vi "FTW-Test-Expressions-Booleanish.vi"() -> (0 "error out":errorcluster)   [LabVIEW 2014]
uses:
  src/core/error/FTW-ERR-ExceptionType.ctl
  src/core/expression/FTW-Expr-BooleanExpressionResult.ctl
  src/core/error/FTW-ERR-ThrowError.vi
  src/core/error/FTW-ERR-NoErrorConstant.vi
  src/core/error/FTW-ERR-CallChain.vi
  src/core/string/FTW-STR-ReplaceWhitespace.vi
  src/core/regex/FTW-Regex.lvclass
panel:
  out "String":string
  out "Array":string[](array[string])
  out "Results":T3(array[cluster])
  out "Lexicon":string="$test == true || $b == false && $c == false"
  out "Capture Groups":string[](array[string])
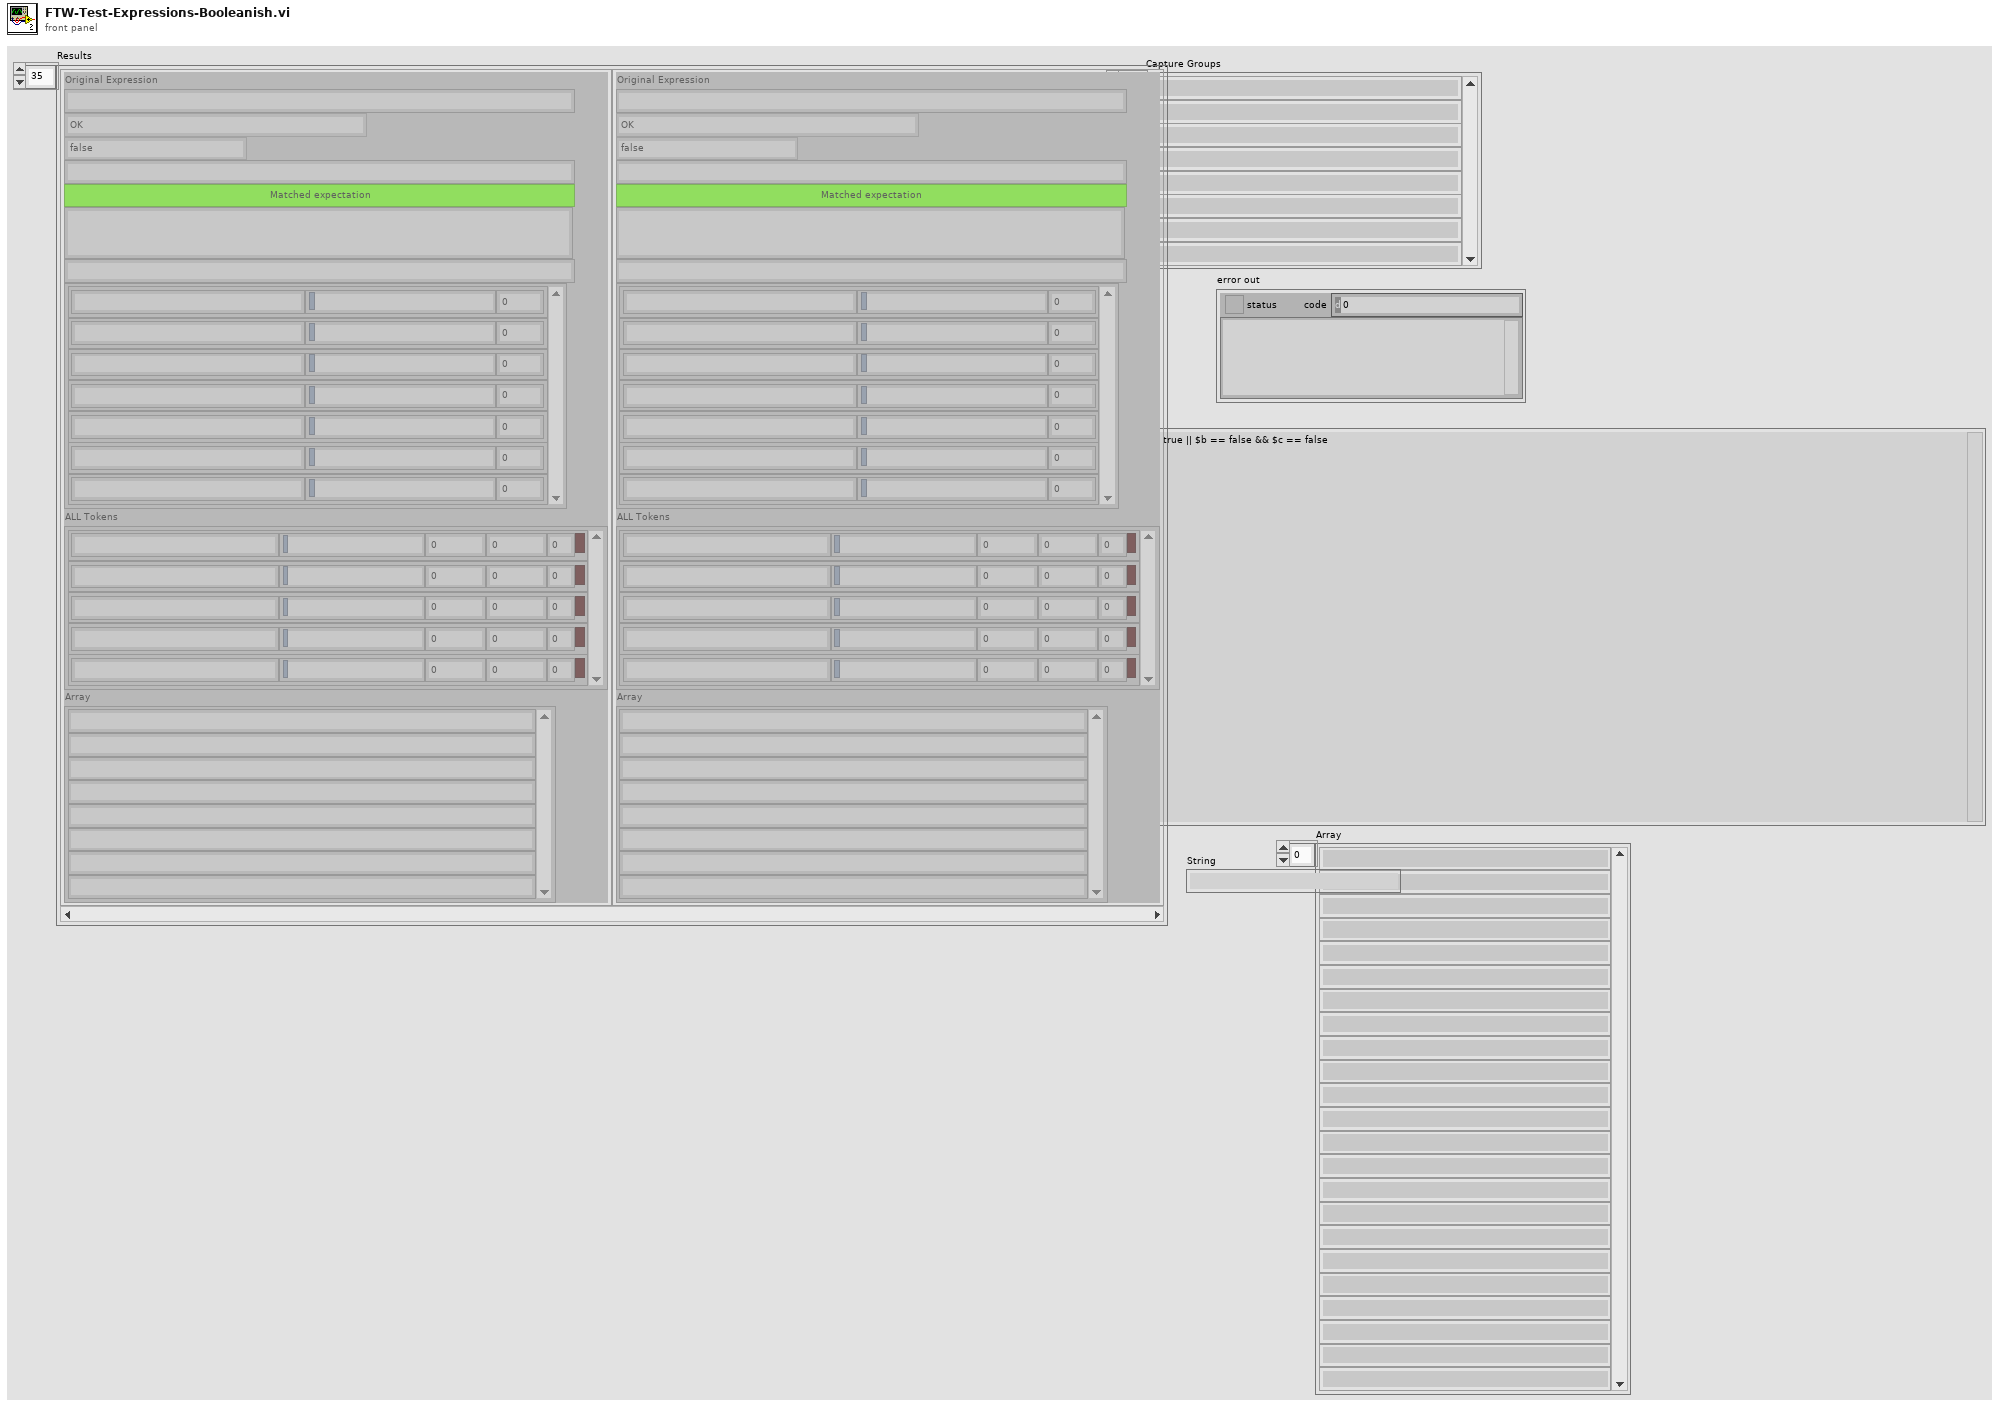
[diagram p1: front panel]
types:
  T1 = typedef "FTW-ERR-ExceptionType.ctl" = enum16{"OK", "Info", "Warning", "Error"}
  T2 = typedef "FTW-Expr-BooleanExpressionResult.ctl" = enum16{"false", "true", "inconclusive"}
  T3 = cluster{"Original Expression":string, "Expression Validity Expectation":T1, "Result":T2, "Expectation":string, "Expectation satisfied?":bool, "Error":string, "Final JSON":string, "Parsed Expression":cluster{string, string, "start_pos":i32}[], "ALL Tokens":cluster{string, string, "prev_pos":i32, "curr_pos":i32, "scope_level":i32, "trimmed?":bool}[], "Array":string[]}[]
  T4 = cluster{"Expression":string, "Expectation":string, "Expression Check":T1, "Value Expectation":T2}[]
  T5 = cluster{"op":cluster{"token":string, "value":string, "subj_start":i32}, "Precedence":i32, "Scope Depth":i32}[]
  T6 = cluster{"token":string, "value":string, "subj_start":i32}[]
  T7 = cluster{"callout_id":i32, "subject_current_pos":i32, "subject_start_match_pos":i32, "cap_top":i32, "cap_last":i32, "patt_pos":i32, "callout_name_index":i32, "callout_name_length":i32}[]
  T8 = cluster{"Text":string, "Expression":string, "Previous Subject Position":i32}
  T9 = cluster{"Text":string, "Expression":string, "Previous Subject Position":i32}[]
  T10 = cluster{cluster{"Text":string, "Expression":string, "Previous Subject Position":i32}, "Precedence":i32, i32}
  T11 = cluster{"op":cluster{"token":string, "value":string, "subj_start":i32}, "Precedence":i32, "Scope Depth":i32}
  T12 = cluster{"token":string, "value":string, "subj_start":i32}
  T13 = cluster{cluster{"Text":string, "Expression":string, "Previous Subject Position":i32}, "default value 1":i32, "Current Scope Depth":i32}
  T14 = cluster{"Text":string, "Expression":string, "subject_current_pos":i32, "Previous Subject Position":i32, "Current Scope Depth":i32, bool}
  T15 = typedef "FTW-JSON-Type.ctl" = enum8{"Not Found", "Object", "Array", "String", "Number", "Boolean", "null"}
  T16 = cluster{"Expression":string, "Expression Check":T1, "Result":T2, "Expectation":string, bool, "source":string, "JSON String (UTF-8)":string, "Reverse Polish Notation Token Stack":cluster{"token":string, "value":string, "subj_start":i32}[], cluster{"Text":string, "Expression":string, "subject_current_pos":i32, "Previous Subject Position":i32, "Current Scope Depth":i32, bool}[], "Try Paths":string[]}
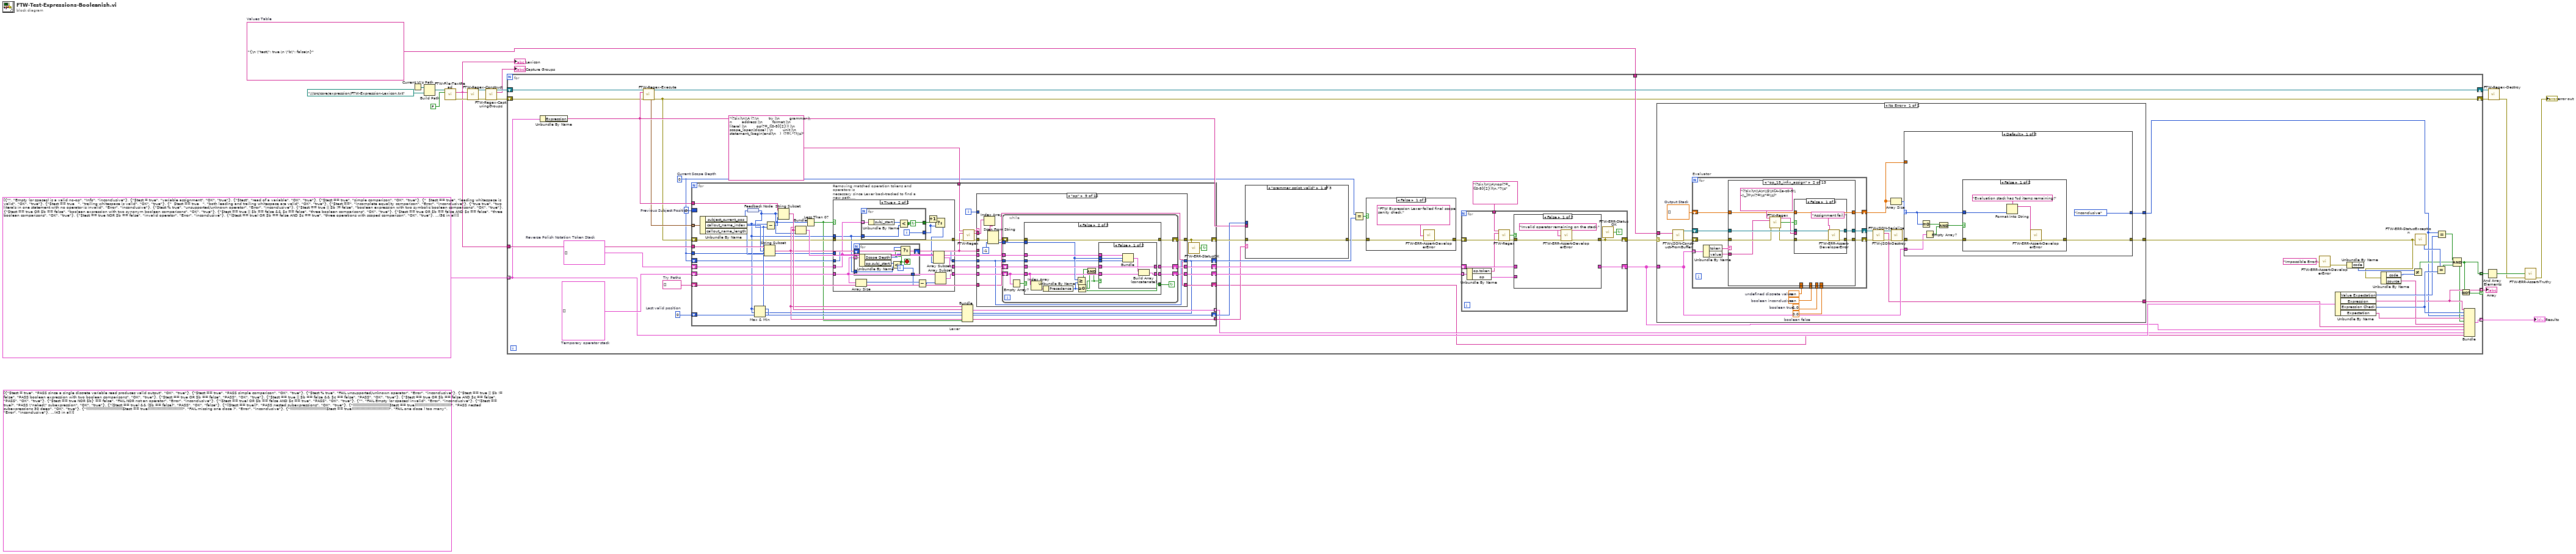
[diagram p0: block diagram]
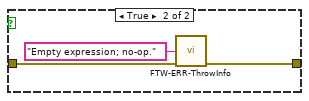
[diagram p2: hidden frame]
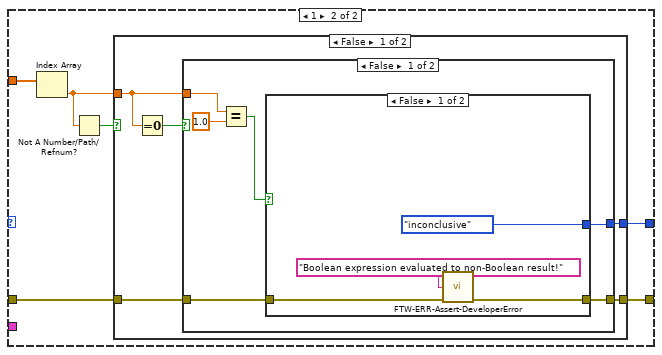
[diagram p3: hidden frame]
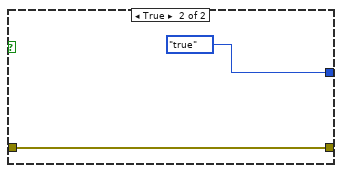
[diagram p4: hidden frame]
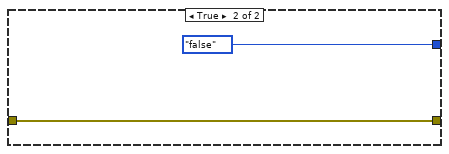
[diagram p5: hidden frame]
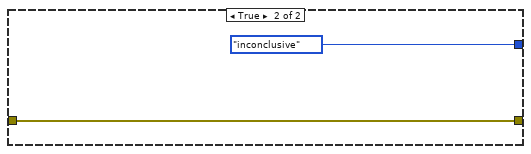
[diagram p6: hidden frame]
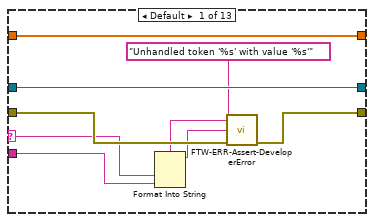
[diagram p7: hidden frame]
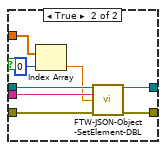
[diagram p8: hidden frame]
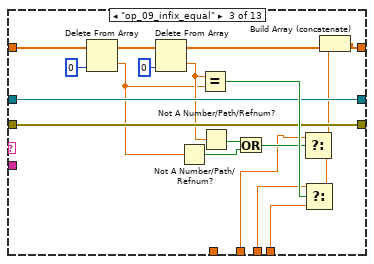
[diagram p9: hidden frame]
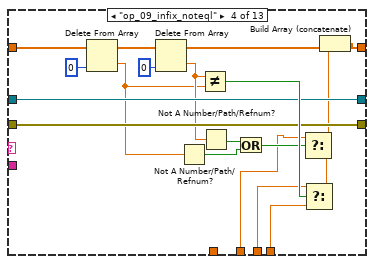
[diagram p10: hidden frame]
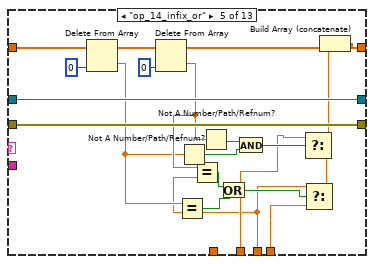
[diagram p11: hidden frame]
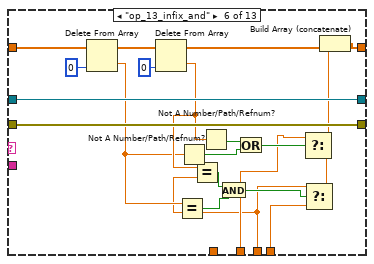
[diagram p12: hidden frame]
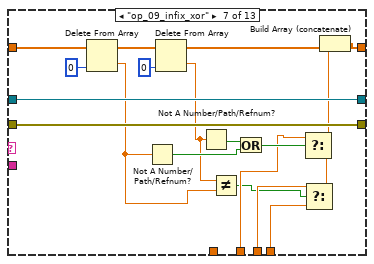
[diagram p13: hidden frame]
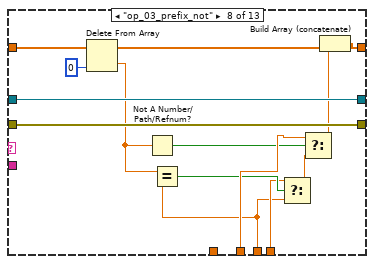
[diagram p14: hidden frame]
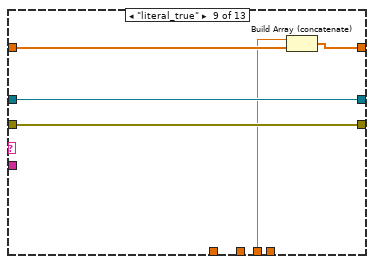
[diagram p15: hidden frame]
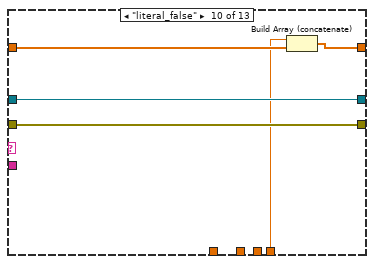
[diagram p16: hidden frame]
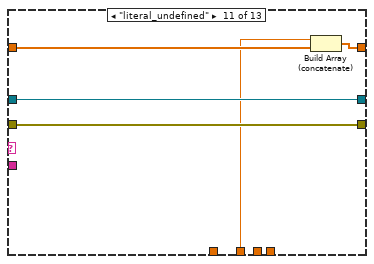
[diagram p17: hidden frame]
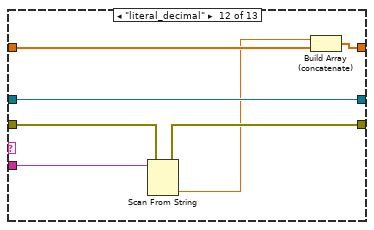
[diagram p18: hidden frame]
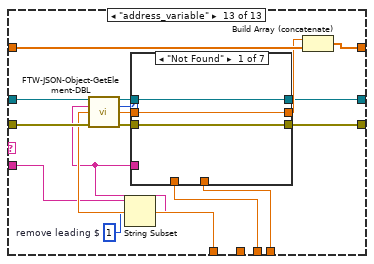
[diagram p19: hidden frame]
diagram:
  (unwired) T4 [{"Expression"="$test = true", "Expectation"="PASS since a single discrete variable read produces valid output", "Expression Check"=enum."OK", "Value Expectation"=enum."true"}, {"Expression"="$test == true", "Expectation"="PASS simple comparison", "Expression Check"=enum."OK", "Value Expectation"=enum."true"}, {"Expression"="$test % true", "Expectation"="FAIL unsupported/unknown operator", "Expression Check"=enum."Error", "Value Expectation"=enum."inconclusive"}, {"Expression"="$test == true || $b != false", "Expectation"="PASS boolean expression with two boolean comparisons", "Expression Check"=enum."OK", "Value Expectation"=enum."true"}, {"Expression"="$test == true OR $b == false", "Expectation"="PASS", "Expression Check"=enum."OK", "Value Expectation"=enum."true"}, {"Expression"="$test == true || $b == false && $c == false", "Expectation"="PASS", "Expression Check"=enum."OK", "Value Expectation"=enum."true"}, {"Expression"="$test == true OR $b == false AND $c == false", "Expectation"="PASS", "Expression Check"=enum."OK", "Value Expectation"=enum."true"}, {"Expression"="$test == true NOR $b} == false", "Expectation"="FAIL NOR not an operator", "Expression Check"=enum."Error", "Value Expectation"=enum."inconclusive"}, {"Expression"="($test == true) OR $b == false AND $c == true", "Expectation"="PASS", "Expression Check"=enum."OK", "Value Expectation"=enum."true"}, {"Expression"="", "Expectation"="FAIL Empty (or spaces) invalid", "Expression Check"=enum."Error", "Value Expectation"=enum."inconclusive"}, {"Expression"="($test == true)", "Expectation"="PASS \"naked\" subexpression", "Expression Check"=enum."OK", "Value Expectation"=enum."true"}, {"Expression"="($test == true) && ($b == false)", "Expectation"="PASS", "Expression Check"=enum."OK", "Value Expectation"=enum."false"}, {"Expression"="(($test == true))", "Expectation"="PASS nested subexpressions", "Expression Check"=enum."OK", "Value Expectation"=enum."true"}, {"Expression"="(((((((((((((((((((((((((((((($test == true))))))))))))))))))))))))))))))", "Expectation"="PASS nested subexpressions 30 deep", "Expression Check"=enum."OK", "Value Expectation"=enum."true"}, {"Expression"="(((((((((((((((((((((((((((((($test == true)))))))))))))))))))))))))))))", "Expectation"="FAIL missing one close )", "Expression Check"=enum."Error", "Value Expectation"=enum."inconclusive"}, {"Expression"="(((((((((((((((((((((((((((((($test == true)))))))))))))))))))))))))))))))", "Expectation"="FAIL one close ) too many", "Expression Check"=enum."Error", "Value Expectation"=enum."inconclusive"}, {"Expression"="true", "Expectation"="PASS plain constant", "Expression Check"=enum."OK", "Value Expectation"=enum."true"}, {"Expression"="False", "Expectation"="PASS plain constant", "Expression Check"=enum."OK", "Value Expectation"=enum."false"}, {"Expression"="ALWAYS AND NEVER", "Expectation"="PASS expression of two boolexpr constants", "Expression Check"=enum."OK", "Value Expectation"=enum."inconclusive"}, {"Expression"="ALWAYS XOR NEVER", "Expectation"="PASS expression of two boolexpr constants", "Expression Check"=enum."OK", "Value Expectation"=enum."inconclusive"}, {"Expression"="(true == true) AND (true EQUALS true) AND (true IS true)", "Expectation"="PASS testing equality operators", "Expression Check"=enum."OK", "Value Expectation"=enum."true"}, {"Expression"="(true != false) AND (true IS NOT false) AND (true <> false)", "Expectation"="PASS testing inequality operators", "Expression Check"=enum."OK", "Value Expectation"=enum."true"}, {"Expression"="(always AND never) XOR (never AND always)", "Expectation"="PASS compound expression of boolexpr constants", "Expression Check"=enum."OK", "Value Expectation"=enum."false"}, {"Expression"="$A==$B", "Expectation"="PASS compare two variables to each other", "Expression Check"=enum."OK", "Value Expectation"=enum."inconclusive"}, {"Expression"="$a!=$b", "Expectation"="PASS since this is a synonym for XOR", "Expression Check"=enum."OK", "Value Expectation"=enum."inconclusive"}, {"Expression"="$A AND $B", "Expectation"="PASS assuming, variables are boolexpr states", "Expression Check"=enum."OK", "Value Expectation"=enum."inconclusive"}, {"Expression"="$a IS true for 3 sec", "Expectation"="SKIP PASS simple timer test", "Expression Check"=enum."OK", "Value Expectation"=enum."inconclusive"}, {"Expression"="$a IS true for 3min", "Expectation"="SKIP PASS no space between timer value and unit", "Expression Check"=enum."OK", "Value Expectation"=enum."inconclusive"}, {"Expression"="$a IS true for 3", "Expectation"="SKIP FAIL no timer units", "Expression Check"=enum."OK", "Value Expectation"=enum."inconclusive"}, {"Expression"="$a IS true   for minute", "Expectation"="SKIP FAIL no timer value", "Expression Check"=enum."OK", "Value Expectation"=enum."inconclusive"}, {"Expression"="$a == true || $b AND $c", "Expectation"="PASS", "Expression Check"=enum."OK", "Value Expectation"=enum."inconclusive"}, {"Expression"="alwaysornever", "Expectation"="FAIL no word boundary on neither operator nor constants", "Expression Check"=enum."OK", "Value Expectation"=enum."inconclusive"}, {"Expression"="always||never", "Expectation"="PASS even though no spaces, the symbolic operator makes a word boundary", "Expression Check"=enum."OK", "Value Expectation"=enum."inconclusive"}, {"Expression"="(($a&&$b) OR ($c&&$d)) AND (($e&&$f) OR ($g&&$h))", "Expectation"="PASS compound expression", "Expression Check"=enum."OK", "Value Expectation"=enum."inconclusive"}, {"Expression"="$a (AND $b)", "Expectation"="FAIL improper placement of parentheses", "Expression Check"=enum."OK", "Value Expectation"=enum."inconclusive"}, {"Expression"="($a)($b)", "Expectation"="FAIL no operator between scopes", "Expression Check"=enum."OK", "Value Expectation"=enum."inconclusive"}, {"Expression"="($a)                   or                 ($b)", "Expectation"="PASS goofy amount of space", "Expression Check"=enum."OK", "Value Expectation"=enum."inconclusive"}, {"Expression"="NOT ALWAYS", "Expectation"="PASS the inversion of a boolexpr constant", "Expression Check"=enum."OK", "Value Expectation"=enum."inconclusive"}, {"Expression"="NOT $a || $b", "Expectation"="PASS even though it could use some parentheses for clarity, this is valid", "Expression Check"=enum."OK", "Value Expectation"=enum."inconclusive"}, {"Expression"="NOT ($a || $b)", "Expectation"="PASS", "Expression Check"=enum."OK", "Value Expectation"=enum."inconclusive"}, {"Expression"="(NOT $a) || $b", "Expectation"="PASS", "Expression Check"=enum."OK", "Value Expectation"=enum."inconclusive"}, {"Expression"="$a && !$b", "Expectation"="PASS", "Expression Check"=enum."OK", "Value Expectation"=enum."inconclusive"}, {"Expression"="IMMEDIATELY", "Expectation"="PASS this is a synonym for ALWAYS", "Expression Check"=enum."OK", "Value Expectation"=enum."inconclusive"}]
  w6 = "{\n \"test\": true,\n \"b\": false\n}"  # Values Table
  n1 = Current VI's Path() -> (path=w17:path)
  n2 = Build Path(base path=w17, name or relative path=path "../../../src/core/expression/FTW-Expression-Lexicon.txt" ("path")) -> (appended path=w15:path)
  n3 = call "FTW-File-TextRead.vi"("Filepath"=w15, "Create if doesn't exist?"=FALSE) -> ("Text"=w18:string, "error out"=w19:errorcluster)  [unwired: 11 in, 1 out]
  "Lexicon" <- w18
  n4 = call "FTW-Regex-Construct.vi"("Regular Expression"=w18, "error in"=w19) -> ("Regex"=w13:refnum<class "FTW-Regex.lvclass">, "error out"=w14:errorcluster)  [unwired: 12 in]
  n5 = call "FTW-Regex-CapturingGroups.vi"("Regex"=w13, "error in"=w14) -> ("Regex out"=w21:refnum<class "FTW-Regex.lvclass">, "Capture Groups"=→"Capture Groups":string[], "error out"=w7:errorcluster)  [unwired: 11 in]
  n6 = for {
    tunnel: w18 -> [w69]
    shift-right: [w54] -> w11
    shift-left: w21 -> [w70]
    tunnel: T4 [{"Expression"="", "Expectation"="Empty (or spaces) is a valid no-op", "Expression Check"=enum."Info", "Value Expectation"=enum."inconclusive"}, {"Expression"="$test = true", "Expectation"="variable assignment", "Expression Check"=enum."OK", "Value Expectation"=enum."true"}, {"Expression"="$test", "Expectation"="read of a variable", "Expression Check"=enum."OK", "Value Expectation"=enum."true"}, {"Expression"="$test == true", "Expectation"="simple comparison", "Expression Check"=enum."OK", "Value Expectation"=enum."true"}, {"Expression"="  $test == true", "Expectation"="leading whitespace is valid", "Expression Check"=enum."OK", "Value Expectation"=enum."true"}, {"Expression"="$test == true   ", "Expectation"="trailing whitespace is valid", "Expression Check"=enum."OK", "Value Expectation"=enum."true"}, {"Expression"="  $test == true   ", "Expectation"="both leading and trailing whitespace are valid", "Expression Check"=enum."OK", "Value Expectation"=enum."true"}, {"Expression"="$test ==", "Expectation"="incomplete equality comparison", "Expression Check"=enum."Error", "Value Expectation"=enum."inconclusive"}, {"Expression"="true true", "Expectation"="two literals in one statement with no operator is invalid", "Expression Check"=enum."Error", "Value Expectation"=enum."inconclusive"}, {"Expression"="$test % true", "Expectation"="unsupported/unknown operator", "Expression Check"=enum."Error", "Value Expectation"=enum."inconclusive"}, {"Expression"="$test == true || $b != false", "Expectation"="boolean expression with two symbolic boolean comparisons", "Expression Check"=enum."OK", "Value Expectation"=enum."true"}, {"Expression"="$test == true OR $b == false", "Expectation"="boolean expression with two synonym boolean comparisons", "Expression Check"=enum."OK", "Value Expectation"=enum."true"}, {"Expression"="$test == true || $b == false && $c == false", "Expectation"="three boolean comparisons", "Expression Check"=enum."OK", "Value Expectation"=enum."true"}, {"Expression"="$test == true OR $b == false AND $c == false", "Expectation"="three boolean comparisons", "Expression Check"=enum."OK", "Value Expectation"=enum."true"}, {"Expression"="$test == true NOR $b == false", "Expectation"="invalid operator", "Expression Check"=enum."Error", "Value Expectation"=enum."inconclusive"}, {"Expression"="($test == true) OR $b == false AND $c == true", "Expectation"="three operations with scoped comparison", "Expression Check"=enum."OK", "Value Expectation"=enum."true"}, {"Expression"="$test OR ($test == false)", "Expectation"="variable comparison with subexpression", "Expression Check"=enum."OK", "Value Expectation"=enum."true"}, {"Expression"="($test == true)", "Expectation"="superfluous subexpression", "Expression Check"=enum."OK", "Value Expectation"=enum."true"}, {"Expression"="($test == true) && ($b == false)", "Expectation"="operation on two subexpressions", "Expression Check"=enum."OK", "Value Expectation"=enum."true"}, {"Expression"="(($test == true))", "Expectation"="nested subexpressions", "Expression Check"=enum."OK", "Value Expectation"=enum."true"}, {"Expression"="(((((((((((((((((((((((((((((($test == true))))))))))))))))))))))))))))))", "Expectation"="PASS nested subexpressions 30 deep", "Expression Check"=enum."OK", "Value Expectation"=enum."true"}, {"Expression"="(((((((((((((((((((((((((((((($test == true)))))))))))))))))))))))))))))", "Expectation"="missing one close )", "Expression Check"=enum."Error", "Value Expectation"=enum."inconclusive"}, {"Expression"="(((((((((((((((((((((((((((((($test == true)))))))))))))))))))))))))))))))", "Expectation"="one close ) too many", "Expression Check"=enum."Error", "Value Expectation"=enum."inconclusive"}, {"Expression"="true", "Expectation"="plain constant", "Expression Check"=enum."OK", "Value Expectation"=enum."true"}, {"Expression"="False", "Expectation"="plain constant", "Expression Check"=enum."OK", "Value Expectation"=enum."false"}, {"Expression"="true XOR false", "Expectation"="expression of two boolexpr constants", "Expression Check"=enum."OK", "Value Expectation"=enum."true"}, {"Expression"="(true == true) AND (true EQUALS true) AND (true IS true)", "Expectation"="testing equality operators", "Expression Check"=enum."OK", "Value Expectation"=enum."true"}, {"Expression"="(true != false) AND (true IS NOT false) AND (true <> false)", "Expectation"="testing inequality operators", "Expression Check"=enum."OK", "Value Expectation"=enum."true"}, {"Expression"="(true AND false) XOR (false AND true)", "Expectation"="compound expression of boolexpr constants", "Expression Check"=enum."OK", "Value Expectation"=enum."false"}, {"Expression"="$A==$B", "Expectation"="compare two variables to each other", "Expression Check"=enum."OK", "Value Expectation"=enum."inconclusive"}, {"Expression"="$a!=$b", "Expectation"="synonym for XOR", "Expression Check"=enum."OK", "Value Expectation"=enum."inconclusive"}, {"Expression"="$A AND $B", "Expectation"="AND two variables", "Expression Check"=enum."OK", "Value Expectation"=enum."inconclusive"}, {"Expression"="$test == ture", "Expectation"="common misspelling of \"true\" is invalid", "Expression Check"=enum."Error", "Value Expectation"=enum."inconclusive"}, {"Expression"="%test == flase", "Expectation"="common misspelling of \"false\" is invalid", "Expression Check"=enum."Error", "Value Expectation"=enum."inconclusive"}, {"Expression"="$test == tru", "Expectation"="incomplete literal \"true\"", "Expression Check"=enum."Error", "Value Expectation"=enum."inconclusive"}, {"Expression"="$test == truee", "Expectation"="extra 'e' in literal \"true\"", "Expression Check"=enum."Error", "Value Expectation"=enum."inconclusive"}, {"Expression"="$test == true!", "Expectation"="unary operator in wrong location", "Expression Check"=enum."Error", "Value Expectation"=enum."inconclusive"}, {"Expression"="$a == true || $b AND $c", "Expectation"="mix of symbolic and synonym operators", "Expression Check"=enum."OK", "Value Expectation"=enum."inconclusive"}, {"Expression"="falseortrue", "Expectation"="invalid without word boundary between operator and literals", "Expression Check"=enum."Error", "Value Expectation"=enum."inconclusive"}, {"Expression"="false||true", "Expectation"="even though no spaces, the symbolic operator makes a word boundary", "Expression Check"=enum."OK", "Value Expectation"=enum."true"}, {"Expression"="(($a&&$b) OR ($c&&$d)) AND (($e&&$f) OR ($g&&$h))", "Expectation"="compound scoped expression", "Expression Check"=enum."OK", "Value Expectation"=enum."inconclusive"}, {"Expression"="$a (AND $b)", "Expectation"="improper placement of parentheses", "Expression Check"=enum."Error", "Value Expectation"=enum."inconclusive"}, {"Expression"="($a)($b)", "Expectation"="no operator between scopes", "Expression Check"=enum."Error", "Value Expectation"=enum."inconclusive"}, {"Expression"="($a)                   or                 ($b)", "Expectation"="goofy but valid amount of space", "Expression Check"=enum."OK", "Value Expectation"=enum."false"}, {"Expression"="NOT $a || $b", "Expectation"="valid, but could use some parentheses for clarity, since precedence applies to first operand and not the result of the operation", "Expression Check"=enum."OK", "Value Expectation"=enum."false"}, {"Expression"="$b || NOT $a", "Expectation"="valid", "Expression Check"=enum."OK", "Value Expectation"=enum."false"}, {"Expression"="$b||!$a", "Expectation"="could use some whitespace, but valid use of symbolic operators", "Expression Check"=enum."OK", "Value Expectation"=enum."false"}, {"Expression"="NOT ($a || $b)", "Expectation"="valid", "Expression Check"=enum."OK", "Value Expectation"=enum."true"}, {"Expression"="(NOT $a) || $b", "Expectation"="valid", "Expression Check"=enum."OK", "Value Expectation"=enum."false"}, {"Expression"="!($a||$b)", "Expectation"="valid", "Expression Check"=enum."OK", "Value Expectation"=enum."true"}, {"Expression"="$a && !$b", "Expectation"="valid", "Expression Check"=enum."OK", "Value Expectation"=enum."inconclusive"}, {"Expression"="! ($test = false)", "Expectation"="assignment in the middle of a statement", "Expression Check"=enum."OK", "Value Expectation"=enum."true"}, {"Expression"="$b | true", "Expectation"="unsupported operator `|`", "Expression Check"=enum."Error", "Value Expectation"=enum."inconclusive"}, {"Expression"="$b & true", "Expectation"="unsupported operator `&`", "Expression Check"=enum."Error", "Value Expectation"=enum."inconclusive"}, {"Expression"="$b IS NOT true", "Expectation"="inequality on boolean", "Expression Check"=enum."OK", "Value Expectation"=enum."true"}, {"Expression"="$b IS NOT NOT false", "Expectation"="inequality on inverted boolean", "Expression Check"=enum."OK", "Value Expectation"=enum."true"}] -> [w52] mode=indexing
    tunnel: [w53] -> w10 mode=indexing
    tunnel: [w31] -> w9 mode=indexing
    tunnel: w6 -> [w41]
    shift-right: [w39] -> w5
    shift-left: w7 -> [w43]
    tunnel: [w32] -> w4 mode=indexing if=w30
    w27 = 0  # Previous Subject Position
    w29 = string[] []  # Try Paths
    w57 = 0  # Last valid position
    w23 = 0  # Current Scope Depth
    w66 = T5 []  # Temporary operator stack
    w67 = T6 []  # Reverse Polish Notation Token Stack
    n7 = Unbundle By Name(w52) -> ("Expression"=w51:string)
    n8 = call "FTW-Regex-Execute.vi"("Regex"=w70, "Subject String"=w51, "error in"=w43) -> ("Regex out"=w54:refnum<class "FTW-Regex.lvclass">, "Callouts"=w40:T7, "error out"=w39:errorcluster)  [unwired: 7 in, 3 out]
    n9 = for "Lexer" {
      tunnel: "(?six)\n\\A (?:\n        try |\n        grammar |\n        address |\n        format |\n        literal |\n        op(?=_([0-9]{2})) |\n        scope_(open|close) | \n        unit |\n        statement_(begin|end)\n   )  (?=(.*?)\\z)" -> [w428]
      shift-right: [w425] -> w58
      shift-left: w67 -> [w403]
      shift-right: [w423] -> w60
      shift-left: w39 -> [w401]
      shift-right: [w421] -> w65
      shift-left: w66 -> [w404]
      shift-right: [w393] -> w63
      shift-left: w23 -> [w397]
      tunnel: w40 -> [w418] mode=indexing
      tunnel: w51 -> [w420]
      tunnel: [w411] -> w42 mode=indexing
      shift-right: [w416] -> w56
      shift-left: w57 -> [w417]
      tunnel: [w409] -> w55
      tunnel: w69 -> [w415]
      shift-right: [w407] -> w28
      shift-left: w29 -> [w408]
      border: w27 -> [_]
      tunnel: w23 -> [w395]
      i -> [w419]
      stop <- w422 continue-if-true
      n10 = Unbundle By Name(w418) -> ("subject_current_pos"=w398:i32, "callout_name_index"=w414:i32, "callout_name_length"=w413:i32)
      n11 = feedback-in #1(w398) -> ()
      n12 = feedback #1() -> (w406:i32)
      n13 = Max & Min(x=w398, y=w417) -> (max(x,y)=w416:i32)  [unwired: 1 out]
      n14 = String Subset(string=w415, offset (0)=w414, length (rest)=w413) -> (substring=w409:string)
      n15 = Subtract(x=w398, y=w406) -> (x-y=w405:i32)
      n16 = String Subset(string=w420, offset (0)=w406, length (rest)=w405) -> (substring=w410:string)
      n17 = Bundle("Text"=w409, "Expression"=w410, "Previous Subject Position"=w406) -> (w412:T8)  [unwired: 1 in]
      n18 = Less Than 0?(x=w405) -> (x < 0?=w394:bool)
      n19 = case "Removing matched operation tokens and operators is \nnecessary since Lexer back-tracked to find a new path,\nnot having found complete grammar of a valid expression" shown="True" w394 {
        tunnel: w404 -> [w431 w436]
        tunnel: w403 -> [w432 w446]
        tunnel: [w430 w447] -> w402
        tunnel: w401 -> [w430 w447]
        tunnel: [w432 w445] -> w400
        tunnel: [w431 w444] -> w399
        tunnel: w398 -> [_ w443]
        tunnel: w397 -> [w429 w437]
        tunnel: [w429 w442] -> w396
        tunnel: w395 -> [_ _]
        frame False {
        }
        frame True {
          n20 = for {
            tunnel: w436 -> [w455] mode=indexing
            tunnel: w443 -> [w453]
            shift-right: [w450] -> w442
            shift-left: w437 -> [w451]
            tunnel: [w448] -> w433
            i -> [w448]
            stop <- w449 stop-if-true
            n21 = Unbundle By Name(w455) -> ("Scope Depth"=w452:i32, "op.subj_start"=w454:i32)
            n22 = Less?(x=w454, y=w453) -> (x < y?=w449:bool)
            n23 = Select(t=w451, s=w449, f=w452) -> (s? t:f=w450:i32)
          }
          n24 = Array Size(array=w436) -> (size(s)=w435:i32)
          n25 = for {
            tunnel: w446 -> [w460] mode=indexing
            tunnel: w443 -> [w458]
            tunnel: [w457] -> w439
            tunnel: [w456] -> w441
            i -> [w457]
            stop <- w456 continue-if-true
            n26 = Unbundle By Name(w460) -> ("subj_start"=w459:i32)
            n27 = Less?(x=w459, y=w458) -> (x < y?=w456:bool)
          }
          n28 = Subtract(x=w435, y=w433) -> (x-y=w434:i32)
          n29 = Increment(x=w439) -> (x+1=w438:i32)
          n30 = Select(t=w438, s=w441, f=w439) -> (s? t:f=w440:i32)
          n31 = Array Subset(array=w446, length=w440) -> (w445:T6)  [unwired: 1 in]
          n32 = Array Subset(array=w436, length=w434) -> (w444:T5)  [unwired: 1 in]
        }
      }
      n33 = call "FTW-Regex.vi"("Regular Expression"=w428, "Input String"=w409, "error in"=w402) -> ("Match"=w427:string, "Submatches"=w426:string[], "error out"=w424:errorcluster)  [unwired: 8 in, 2 out]
      n34 = case shown="\"op\"" w427 {
        tunnel: w426 -> [_ _ _ _ w493 _ _ _ w568 _ _ _]
        tunnel: w412 -> [_ w476 w483 _ _ _ w510 w520 w569 _ _ _]
        tunnel: w400 -> [w467 w475 w482 w488 w497 w504 w513 w524 w573 w629 w634 w639]
        tunnel: [w467 w474 w481 w488 w497 w504 w513 w522 w574 w629 w634 w639] -> w425
        tunnel: [w468 w473 w480 w487 w496 w501 w514 w519 w571 w630 w635 w640] -> w423
        tunnel: w424 -> [w469 w473 w480 w487 w496 w501 w514 w518 w578 w630 w635 w640]
        tunnel: [w466 w472 w479 w486 w495 w503 w511 w521 w570 w628 w633 w638] -> w421
        tunnel: w399 -> [w466 w472 w479 w486 w495 w503 w512 w523 w575 w628 w633 w638]
        tunnel: w409 -> [w463 _ _ _ w489 w498 _ _ _ _ _ _]
        tunnel: w396 -> [w462 w471 w478 w485 w494 w502 w508 w517 w566 w627 w632 w637]
        tunnel: [w462 w471 w478 w485 w494 w502 w507 w516 w566 w627 w632 w637] -> w393
        tunnel: w419 -> [_ _ _ _ _ _ _ _ _ _ _ _]
        tunnel: w408 -> [w461 w470 w477 w484 w491 w500 w505 w515 w565 w626 w631 w636]
        tunnel: [w461 w470 w477 w484 w490 w499 w505 w515 w565 w626 w631 w636] -> w407
        frame Default {
          n35 = Format Into String(format string="Bug in the FTW evaluation compiler! Unknown token: \"%s\"" ("Reason this error should never happen"), w463) -> (resulting string=w464:string)  [unwired: 2 in, 1 out]
          n36 = call "FTW-ERR-Assert-DeveloperError.vi"("Reason this error should never happen"=w464, "error in"=w469) -> ("error out"=w468:errorcluster)  [unwired: 13 in]
        }
        frame "literal" {
          n37 = Build Array (concatenate)(w475, w476) -> (w474:T9)
        }
        frame "address" {
          n38 = Build Array (concatenate)(w482, w483) -> (w481:T9)
        }
        frame "format" {
          # "Format matches are included in the\ncallout array purely to maintain match position\nof tokens."
        }
        frame "try" {
          # "Format matches are included in the\ncallout array purely to maintain match position\nof tokens."
          n39 = Index Array(array=w493) -> (element=→"String":string)  [unwired: 1 in]
          n40 = Build Array (concatenate)(w491, w489) -> (w490:string[])
        }
        frame "grammar" {
          # "Grammar matches are included in the\ncallout array in order to maintain match position\nof tokens and to validate grammar."
          n41 = Build Array (concatenate)(w500, w498) -> (w499:string[])
        }
        frame "scope_open" {
          w506 = -1  # Precedence
          n42 = Increment(x=w508) -> (x+1=w507:i32)
          n43 = Bundle(w510, "Precedence"=w506, w507) -> (w509:T10)  [unwired: 1 in]
          n44 = Build Array (concatenate)(w509, w512) -> (w511:T5)
        }
        frame "scope_close" {
          n45 = while {
            shift-right: [w530] -> w519
            shift-left: w518 -> [w531]
            shift-right: [w539] -> w522
            shift-left: w524 -> [w538]
            shift-right: [w537] -> w521
            shift-left: w523 -> [w536]
            tunnel: w520 -> [_]
            shift-right: [w527] -> w516
            shift-left: w517 -> [w526]
            stop <- w528 continue-if-true
            n46 = Delete From Array(array=w536, index=0) -> (deleted portion=w534:T11, array with subset deleted=w532:T5)  [unwired: 1 in]
            n47 = Unbundle By Name(w534) -> ("Scope Depth"=w525:i32, "op"=w529:T12, "op.token"=w533:string)
            n48 = case shown="Default" w533 {
              tunnel: [w548 w560] -> w539
              tunnel: w538 -> [w547 w560]
              tunnel: [w544 w559] -> w537
              tunnel: w532 -> [w544 w559]
              tunnel: w531 -> [w545 w555]
              tunnel: [w542 w554] -> w530
              tunnel: w529 -> [w546 _]
              tunnel: [w541 _] -> w528
              tunnel: [w540 w558] -> w527
              tunnel: w526 -> [w540 w556]
              tunnel: w525 -> [_ w557]
              frame Default {
                n49 = Empty Array?(array=w544) -> (empty?=w543:bool)
                n50 = case shown="True" w543 {
                  tunnel: w545 -> [w549 w552]
                  tunnel: [w549 w550] -> w542
                  frame False {
                  }
                  frame True {
                    n51 = call "FTW-ERR-Assert-DeveloperError.vi"("Reason this error should never happen"="Mismatched scope", "error in"=w552) -> ("error out"=w550:errorcluster)  [unwired: 13 in]
                  }
                }
                n52 = Build Array (concatenate)(w547, w546) -> (w548:T6)
                n53 = call "FTW-ERR-StatusOK.vi"("error to check"=w542) -> ("Status OK?"=w541:bool)
              }
              frame "scope_open" {
                # "Found it the matching\nscope_open token;\nsilently discard it."
                n54 = Not Equal?(x=w557, y=w556) -> (x != y?=w553:bool)
                n55 = case shown="True" w553 {
                  tunnel: w555 -> [w561 w564]
                  tunnel: [w561 w562] -> w554
                  frame False {
                  }
                  frame True {
                    n56 = call "FTW-ERR-Assert-DeveloperError.vi"("Reason this error should never happen"="Mismatched scope level", "error in"=w564) -> ("error out"=w562:errorcluster)  [unwired: 13 in]
                  }
                }
                n57 = Decrement(x=w556) -> (x-1=w558:i32)
              }
            }
          }
        }
        frame "op" {
          n58 = Index Array(array=w568) -> (element=w567:string)  [unwired: 1 in]
          n59 = Scan From String(input string=w567, error in=w578, default 1=-1 ("default value 1")) -> (error out=w572:errorcluster, output 1=w576:i32)  [unwired: 2 in, 2 out]
          n60 = while {
            tunnel: w576 -> [w584]
            shift-right: [w580] -> w571
            shift-left: w572 -> [w579]
            shift-right: [w589] -> w574
            shift-left: w573 -> [w588]
            shift-right: [w587] -> w570
            shift-left: w575 -> [w586]
            tunnel: w569 -> [w585]
            tunnel: w566 -> [w583]
            stop <- w581 continue-if-true
            n61 = Empty Array?(array=w586) -> (empty?=w582:bool)
            n62 = case shown="False" w582 {
              tunnel: [w598 w611] -> w589
              tunnel: w588 -> [w598 w610]
              tunnel: [w597 w609] -> w587
              tunnel: w586 -> [w596 w605]
              tunnel: w585 -> [w595 w608]
              tunnel: w584 -> [w594 w607]
              tunnel: w583 -> [w593 w606]
              tunnel: [FALSE w599] -> w581
              tunnel: [w590 w603] -> w580
              tunnel: w579 -> [w590 w603]
              frame True {
                n63 = Bundle(w595, "default value 1"=w594, "Current Scope Depth"=w593) -> (w592:T13)  [unwired: 1 in]
                n64 = Build Array (concatenate)(w592, w596) -> (w597:T5)
              }
              frame False {
                n65 = Index Array(array=w605) -> (element=w604:T11)  [unwired: 1 in]
                n66 = Unbundle By Name(w604) -> ("Precedence"=w602:i32)
                n67 = Greater Or Equal?(x=w607, y=w602) -> (x >= y?=w601:bool)
                n68 = Greater Or Equal To 0?(x=w602) -> (x >= 0?=w600:bool)
                n69 = And(x=w601, y=w600) -> (x .and. y?=w599:bool)
                n70 = case shown="False" w599 {
                  tunnel: [w618 w624] -> w611
                  tunnel: w610 -> [w618 w625]
                  tunnel: [w616 w619] -> w609
                  tunnel: w605 -> [w617 w620]
                  tunnel: w608 -> [w615 _]
                  tunnel: w607 -> [w614 _]
                  tunnel: w606 -> [w612 _]
                  frame False {
                    n71 = Bundle(w615, "default value 1"=w614, "Current Scope Depth"=w612) -> (w613:T13)  [unwired: 1 in]
                    n72 = Build Array (concatenate)(w613, w617) -> (w616:T5)
                  }
                  frame True {
                    n73 = Delete From Array(array=w620, index=0) -> (deleted portion=w622:T11, array with subset deleted=w619:T5)  [unwired: 1 in]
                    n74 = Unbundle(w622) -> ("op"=w621:T12)  [unwired: 2 out]
                    n75 = Build Array (concatenate)(w625, w621) -> (w624:T6)
                  }
                }
              }
            }
          }
        }
        frame "unit" {
        }
        frame "statement_begin" {
        }
        frame "statement_end" {
        }
      }
      n76 = Bundle("Text"=w409, "Expression"=w410, "subject_current_pos"=w398, "Previous Subject Position"=w406, "Current Scope Depth"=w393, w394) -> (w411:T14)  [unwired: 1 in]
      n77 = call "FTW-ERR-StatusOK.vi"("error to check"=w423) -> ("Status OK?"=w422:bool)
    }
    n78 = case shown="\"grammar_script_valid\"" w55 {
      tunnel: [w359 w361 w370] -> w59
      tunnel: w60 -> [w359 w362 w369]
      tunnel: w56 -> [_ _ w365]
      tunnel: w51 -> [_ _ w366]
      frame "grammar_script_valid" {
      }
      frame Default {
        n79 = call "FTW-ERR-Assert-DeveloperError.vi"("Reason this error should never happen"="Bogus lexing regex.", "error in"=w362) -> ("error out"=w361:errorcluster)  [unwired: 13 in]
      }
      frame "grammar_script_invalid" {
        n80 = String Subset(string=w366, offset (0)=w365, length (rest)=8 ("length (rest)")) -> (substring=w363:string)
        n81 = Format Into String(format string="Syntax error near character position %d beginning with \"%s\"" ("Error Message"), w365, w363) -> (resulting string=w367:string)  [unwired: 2 in, 1 out]
        n82 = call "FTW-ERR-ThrowGenericError.vi"("Error Message"=w367, "error in"=w369) -> ("error out"=w370:errorcluster)  [unwired: 13 in]
      }
    }
    n83 = Equal?(x=w23, y=w63) -> (x = y?=w62:bool)
    n84 = case shown="False" w62 {
      tunnel: w59 -> [w372 w374]
      tunnel: [w371 w374] -> w61
      frame False {
        n85 = call "FTW-ERR-Assert-DeveloperError.vi"("Reason this error should never happen"="FTW Expression Lexer failed final scope sanity check.", "error in"=w372) -> ("error out"=w371:errorcluster)  [unwired: 13 in]
      }
      frame True {
      }
    }
    n86 = for {
      tunnel: w65 -> [w385] mode=indexing
      shift-right: [w376] -> w33
      shift-left: w61 -> [w384]
      tunnel: "(?six)\n\\A\nop(?=_([0-9]{2}))\n.*?\\z" ("Regular Expression") -> [w383]
      shift-right: [w378] -> w25
      shift-left: w58 -> [w379]
      stop <- w375 continue-if-true
      n87 = Unbundle By Name(w385) -> ("op.token"=w377:string, "op"=w380:T12)
      n88 = call "FTW-Regex.vi"("Regular Expression"=w383, "Input String"=w377, "error in"=w384) -> ("Match Found?"=w382:bool, "error out"=w381:errorcluster)  [unwired: 8 in, 3 out]
      n89 = case shown="False" w382 {
        tunnel: w381 -> [w388 w392]
        tunnel: [w386 w392] -> w376
        tunnel: w380 -> [_ w391]
        tunnel: w379 -> [_ w390]
        tunnel: [_ w389] -> w378
        frame False {
          n90 = call "FTW-ERR-Assert-DeveloperError.vi"("Reason this error should never happen"="Invalid operator remaining on the stack.", "error in"=w388) -> ("error out"=w386:errorcluster)  [unwired: 13 in]
        }
        frame True {
          n91 = Build Array (concatenate)(w390, w391) -> (w389:T6)
        }
      }
      n92 = call "FTW-ERR-StatusOK.vi"("error to check"=w376) -> ("Status OK?"=w375:bool)
    }
    n93 = case shown="No Error" w33 {
      selector: w33 -> [w82 w358]
      tunnel: [w78 w358] -> w24
      tunnel: w25 -> [w76 _]
      tunnel: w41 -> [w83 _]
      tunnel: [w77 FTW-Expr-BooleanExpressionResult."inconclusive" ("Result")] -> w26
      tunnel: [w71 "" ("JSON String (UTF-8)")] -> w22
      frame No Error {
        w84 = nan  # undefined discrete value
        w85 = nan  # boolean inconclusive
        w86 = 1.0  # boolean true
        w87 = 0.0  # boolean false
        w88 = dbl[] []  # Output Stack
        n94 = call "FTW-JSON-Construct-FromBuffer.vi"("JSON String (UTF-8)"=w83, "error in"=w82) -> ("JSON Object"=w89:refnum<data-value>, "error out"=w90:errorcluster)  [unwired: 12 in]
        n95 = for "Evaluator" {
          tunnel: w76 -> [w146] mode=indexing
          shift-right: [w143] -> w80
          shift-left: w88 -> [w144]
          shift-right: [w141] -> w75
          shift-left: w89 -> [w142]
          shift-right: [w139] -> w73
          shift-left: w90 -> [w140]
          tunnel: w87 -> [w138]
          tunnel: w86 -> [w137]
          tunnel: w85 -> [w136]
          tunnel: w84 -> [w135]
          n96 = Unbundle By Name(w146) -> ("token"=w145:string, "value"=w134:string)
          n97 = case shown="\"op_15_infix_assign\"" w145 {
            selector: w145 -> [w148 _ _ _ _ _ _ _ _ _ _ _ _]
            tunnel: w144 -> [w154 w156 w195 w214 w235 w256 w275 w289 w294 w299 w304 w311 w328]
            tunnel: [w154 w156 w189 w208 w230 w251 w270 w287 w293 w298 w303 w310 w327] -> w143
            tunnel: w142 -> [w153 w164 w188 w207 w229 w250 w269 w286 w292 w297 w302 w309 w326]
            tunnel: [w153 w163 w188 w207 w229 w250 w269 w286 w292 w297 w302 w309 w318] -> w141
            tunnel: w140 -> [w152 w161 w187 w206 w228 w249 w268 w285 w291 w296 w301 w307 w325]
            tunnel: [w151 w162 w187 w206 w228 w249 w268 w285 w291 w296 w301 w306 w317] -> w139
            tunnel: w134 -> [w147 w158 _ _ _ _ _ _ _ _ _ w308 w313]
            tunnel: w138 -> [_ _ w179 w198 w222 w243 w262 w278 _ w295 _ _ w315]
            tunnel: w137 -> [_ _ w178 w197 w217 w238 w260 w277 w290 _ _ _ w316]
            tunnel: w136 -> [_ _ w177 w196 w221 w242 w261 w283 _ _ w300 _ _]
            tunnel: w135 -> [_ _ _ _ _ _ _ _ _ _ _ _ w324]
            frame Default {
              n98 = Format Into String(format string="Unhandled token '%s' with value '%s'" ("Reason this error should never happen"), w148, w147) -> (resulting string=w150:string)  [unwired: 2 in, 1 out]
              n99 = call "FTW-ERR-Assert-DeveloperError.vi"("Reason this error should never happen"=w150, "error in"=w152) -> ("error out"=w151:errorcluster)  [unwired: 13 in]
            }
            frame "op_15_infix_assign" {
              n100 = call "FTW-Regex.vi"("Regular Expression"="(?six)\n\\A\n\\$\\K[A-Za-z0-9\\-\\_]+\n(?=\\s*=\\z)", "Input String"=w158, "error in"=w161) -> ("Match"=w157:string, "Match Found?"=w155:bool, "error out"=w160:errorcluster)  [unwired: 8 in, 2 out]
              n101 = case shown="False" w155 {
                tunnel: w164 -> [w168 w176]
                tunnel: [w168 w175] -> w163
                tunnel: [w166 w174] -> w162
                tunnel: w160 -> [w167 w173]
                tunnel: w157 -> [_ w172]
                tunnel: w156 -> [_ w170]
                frame False {
                  n102 = call "FTW-ERR-Assert-DeveloperError.vi"("Reason this error should never happen"="Assignment fail.", "error in"=w167) -> ("error out"=w166:errorcluster)  [unwired: 13 in]
                }
                frame True {
                  n103 = Index Array(array=w170, index=0) -> (element=w169:dbl)
                  n104 = call "FTW-JSON-Object-SetElement-DBL.vi"("JSON Object"=w176, "Key"=w172, "Value"=w169, "error in"=w173) -> ("JSON Object out"=w175:refnum<data-value>, "error out"=w174:errorcluster)  [unwired: 10 in]
                }
              }
            }
            frame "op_09_infix_equal" {
              n105 = Delete From Array(array=w195, index=0) -> (deleted portion=w185:dbl, array with subset deleted=w193:dbl[])  [unwired: 1 in]
              n106 = Delete From Array(array=w193, index=0) -> (deleted portion=w186:dbl, array with subset deleted=w190:dbl[])  [unwired: 1 in]
              n107 = Not A Number/Path/Refnum?(number/path/refnum=w185) -> (NaN/Path/Refnum?=w183:bool)
              n108 = Equal?(x=w186, y=w185) -> (x = y?=w191:bool)
              n109 = Not A Number/Path/Refnum?(number/path/refnum=w186) -> (NaN/Path/Refnum?=w184:bool)
              n110 = Or(x=w184, y=w183) -> (x .or. y?=w182:bool)
              n111 = Select(t=w178, s=w191, f=w179) -> (s? t:f=w181:dbl)
              n112 = Select(t=w177, s=w182, f=w181) -> (s? t:f=w180:dbl)
              n113 = Build Array (concatenate)(w180, w190) -> (w189:dbl[])
            }
            frame "op_09_infix_noteql" {
              n114 = Delete From Array(array=w214, index=0) -> (deleted portion=w204:dbl, array with subset deleted=w212:dbl[])  [unwired: 1 in]
              n115 = Delete From Array(array=w212, index=0) -> (deleted portion=w205:dbl, array with subset deleted=w209:dbl[])  [unwired: 1 in]
              n116 = Not A Number/Path/Refnum?(number/path/refnum=w204) -> (NaN/Path/Refnum?=w202:bool)
              n117 = Not Equal?(x=w205, y=w204) -> (x != y?=w210:bool)
              n118 = Not A Number/Path/Refnum?(number/path/refnum=w205) -> (NaN/Path/Refnum?=w203:bool)
              n119 = Or(x=w203, y=w202) -> (x .or. y?=w201:bool)
              n120 = Select(t=w197, s=w210, f=w198) -> (s? t:f=w200:dbl)
              n121 = Select(t=w196, s=w201, f=w200) -> (s? t:f=w199:dbl)
              n122 = Build Array (concatenate)(w199, w209) -> (w208:dbl[])
            }
            frame "op_14_infix_or" {
              n123 = Delete From Array(array=w235, index=0) -> (deleted portion=w218:dbl, array with subset deleted=w233:dbl[])  [unwired: 1 in]
              n124 = Delete From Array(array=w233, index=0) -> (deleted portion=w219:dbl, array with subset deleted=w231:dbl[])  [unwired: 1 in]
              n125 = Equal?(x=w218, y=w217) -> (x = y?=w216:bool)
              n126 = Not A Number/Path/Refnum?(number/path/refnum=w218) -> (NaN/Path/Refnum?=w226:bool)
              n127 = Equal?(x=w219, y=w217) -> (x = y?=w215:bool)
              n128 = Not A Number/Path/Refnum?(number/path/refnum=w219) -> (NaN/Path/Refnum?=w227:bool)
              n129 = Or(x=w215, y=w216) -> (x .or. y?=w220:bool)
              n130 = And(x=w227, y=w226) -> (x .and. y?=w225:bool)
              n131 = Select(t=w217, s=w220, f=w222) -> (s? t:f=w224:dbl)
              n132 = Select(t=w221, s=w225, f=w224) -> (s? t:f=w223:dbl)
              n133 = Build Array (concatenate)(w223, w231) -> (w230:dbl[])
            }
            frame "op_13_infix_and" {
              n134 = Delete From Array(array=w256, index=0) -> (deleted portion=w239:dbl, array with subset deleted=w254:dbl[])  [unwired: 1 in]
              n135 = Delete From Array(array=w254, index=0) -> (deleted portion=w240:dbl, array with subset deleted=w252:dbl[])  [unwired: 1 in]
              n136 = Equal?(x=w239, y=w238) -> (x = y?=w237:bool)
              n137 = Not A Number/Path/Refnum?(number/path/refnum=w239) -> (NaN/Path/Refnum?=w247:bool)
              n138 = Equal?(x=w240, y=w238) -> (x = y?=w236:bool)
              n139 = Not A Number/Path/Refnum?(number/path/refnum=w240) -> (NaN/Path/Refnum?=w248:bool)
              n140 = And(x=w236, y=w237) -> (x .and. y?=w241:bool)
              n141 = Or(x=w248, y=w247) -> (x .or. y?=w246:bool)
              n142 = Select(t=w238, s=w241, f=w243) -> (s? t:f=w245:dbl)
              n143 = Select(t=w242, s=w246, f=w245) -> (s? t:f=w244:dbl)
              n144 = Build Array (concatenate)(w244, w252) -> (w251:dbl[])
            }
            frame "op_09_infix_xor" {
              n145 = Delete From Array(array=w275, index=0) -> (deleted portion=w258:dbl, array with subset deleted=w273:dbl[])  [unwired: 1 in]
              n146 = Not A Number/Path/Refnum?(number/path/refnum=w258) -> (NaN/Path/Refnum?=w266:bool)
              n147 = Delete From Array(array=w273, index=0) -> (deleted portion=w257:dbl, array with subset deleted=w271:dbl[])  [unwired: 1 in]
              n148 = Not A Number/Path/Refnum?(number/path/refnum=w257) -> (NaN/Path/Refnum?=w267:bool)
              n149 = Not Equal?(x=w257, y=w258) -> (x != y?=w259:bool)
              n150 = Or(x=w267, y=w266) -> (x .or. y?=w265:bool)
              n151 = Select(t=w260, s=w259, f=w262) -> (s? t:f=w264:dbl)
              n152 = Select(t=w261, s=w265, f=w264) -> (s? t:f=w263:dbl)
              n153 = Build Array (concatenate)(w263, w271) -> (w270:dbl[])
            }
            frame "op_03_prefix_not" {
              n154 = Delete From Array(array=w289, index=0) -> (deleted portion=w280:dbl, array with subset deleted=w282:dbl[])  [unwired: 1 in]
              n155 = Not A Number/Path/Refnum?(number/path/refnum=w280) -> (NaN/Path/Refnum?=w281:bool)
              n156 = Equal?(x=w280, y=w277) -> (x = y?=w279:bool)
              n157 = Select(t=w278, s=w279, f=w277) -> (s? t:f=w276:dbl)
              n158 = Select(t=w283, s=w281, f=w276) -> (s? t:f=w284:dbl)
              n159 = Build Array (concatenate)(w284, w282) -> (w287:dbl[])
            }
            frame "literal_true" {
              n160 = Build Array (concatenate)(w290, w294) -> (w293:dbl[])
            }
            frame "literal_false" {
              n161 = Build Array (concatenate)(w295, w299) -> (w298:dbl[])
            }
            frame "literal_undefined" {
              n162 = Build Array (concatenate)(w300, w304) -> (w303:dbl[])
            }
            frame "literal_decimal" {
              n163 = Scan From String(input string=w308, error in=w307) -> (error out=w306:errorcluster, output 1=w305:dbl)  [unwired: 3 in, 2 out]
              n164 = Build Array (concatenate)(w305, w311) -> (w310:dbl[])
            }
            frame "address_variable" {
              w314 = 1  # remove leading $
              n165 = String Subset(string=w313, offset (0)=w314) -> (substring=w312:string)  [unwired: 1 in]
              n166 = call "FTW-JSON-Object-GetElement-DBL.vi"("JSON Object"=w326, "Key"=w312, "Default Value"=w324, "error in"=w325) -> ("JSON Object out"=w319:refnum<data-value>, "JSON Element Type"=w323:T15, "Value"=w320:dbl, "error out"=w322:errorcluster)  [unwired: 8 in]
              n167 = case shown="\"Not Found\"" w323 {
                tunnel: w322 -> [w329 w332 w336 w339 w342 w345 w355]
                tunnel: [w331 w334 w335 w338 w341 w344 w347] -> w321
                tunnel: w320 -> [w331 w334 w335 w338 w341 w344 _]
                tunnel: w319 -> [w330 w333 w337 w340 w343 w346 w354]
                tunnel: [w330 w333 w337 w340 w343 w346 w353] -> w318
                tunnel: [w329 w332 w336 w339 w342 w345 w352] -> w317
                tunnel: w312 -> [_ _ _ _ _ _ w351]
                tunnel: w316 -> [_ _ _ _ _ _ w350]
                tunnel: w315 -> [_ _ _ _ _ _ w348]
                frame "Not Found" {
                }
                frame "null" {
                }
                frame "Object" {
                }
                frame "Array" {
                }
                frame "String" {
                }
                frame "Number" {
                }
                frame "Boolean" {
                  n168 = call "FTW-JSON-Object-GetElement-Bool.vi"("JSON Object"=w354, "Key"=w351, "error in"=w355) -> ("JSON Object out"=w353:refnum<data-value>, "Value"=w349:bool, "error out"=w352:errorcluster)  [unwired: 9 in, 1 out]
                  n169 = Select(t=w350, s=w349, f=w348) -> (s? t:f=w347:dbl)
                }
              }
              n170 = Build Array (concatenate)(w321, w328) -> (w327:dbl[])
            }
          }
        }
        n171 = call "FTW-JSON-Serialize.vi"("JSON Object"=w75, "error in"=w73) -> ("JSON Object out"=w74:refnum<data-value>, "JSON String (UTF-8)"=w71:string, "error out"=w72:errorcluster)  [unwired: 11 in]
        n172 = Array Size(array=w80) -> (size(s)=w81:i32)
        n173 = call "FTW-JSON-Destroy.vi"("JSON Object"=w74, "error in"=w72) -> ("error out"=w79:errorcluster)  [unwired: 13 in]
        n174 = case shown="Default" w81 {
          selector: w81 -> [w93 _]
          tunnel: w79 -> [w98 w110]
          tunnel: [w97 w111] -> w78
          tunnel: w80 -> [_ w112]
          tunnel: [FTW-Expr-BooleanExpressionResult."inconclusive" ("Result") w108] -> w77
          tunnel: w76 -> [w94 _]
          frame Default {
            n175 = Equal To 0?(x=w93) -> (x = 0?=w95:bool)
            n176 = Empty Array?(array=w94) -> (empty?=w92:bool)
            n177 = And(x=w95, y=w92) -> (x .and. y?=w91:bool)
            n178 = case shown="False" w91 {
              tunnel: w98 -> [w103 w106]
              tunnel: [w102 w105] -> w97
              tunnel: w93 -> [w99 _]
              frame False {
                n179 = Format Into String(format string="Evaluation stack has %d items remaining!" ("Reason this error should never happen"), w99) -> (resulting string=w100:string)  [unwired: 2 in, 1 out]
                n180 = call "FTW-ERR-Assert-DeveloperError.vi"("Reason this error should never happen"=w100, "error in"=w103) -> ("error out"=w102:errorcluster)  [unwired: 13 in]
              }
              frame True {
                n181 = call "FTW-ERR-ThrowInfo.vi"("Informational Message"="Empty expression; no-op.", "error in"=w106) -> ("error out"=w105:errorcluster)  [unwired: 13 in]
              }
            }
          }
          frame 1 {
            n182 = Index Array(array=w112) -> (element=w107:dbl)  [unwired: 1 in]
            n183 = Not A Number/Path/Refnum?(number/path/refnum=w107) -> (NaN/Path/Refnum?=w109:bool)
            n184 = case shown="False" w109 {
              tunnel: [w117 w132] -> w111
              tunnel: w110 -> [w116 w132]
              tunnel: [w114 FTW-Expr-BooleanExpressionResult."inconclusive" ("Result")] -> w108
              tunnel: w107 -> [w113 _]
              frame False {
                n185 = Equal To 0?(x=w113) -> (x = 0?=w115:bool)
                n186 = case shown="False" w115 {
                  tunnel: [w122 w131] -> w117
                  tunnel: w116 -> [w123 w131]
                  tunnel: [w118 FTW-Expr-BooleanExpressionResult."false" ("Result")] -> w114
                  tunnel: w113 -> [w121 _]
                  frame False {
                    n187 = Equal?(x=w121, y=1.0) -> (x = y?=w119:bool)
                    n188 = case shown="False" w119 {
                      tunnel: w123 -> [w126 w128]
                      tunnel: [w125 w128] -> w122
                      tunnel: [FTW-Expr-BooleanExpressionResult."inconclusive" ("Result") FTW-Expr-BooleanExpressionResult."true" ("Result")] -> w118
                      frame False {
                        n189 = call "FTW-ERR-Assert-DeveloperError.vi"("Reason this error should never happen"="Boolean expression evaluated to non-Boolean result!", "error in"=w126) -> ("error out"=w125:errorcluster)  [unwired: 13 in]
                      }
                      frame True {
                      }
                    }
                  }
                  frame True {
                  }
                }
              }
              frame True {
              }
            }
          }
        }
      }
      frame Error {
      }
    }
    n190 = call "FTW-ERR-Assert-DeveloperError.vi"("Reason this error should never happen"="Impossible Error") -> ("error out"=w38:errorcluster)  [unwired: 14 in]
    n191 = Unbundle By Name(w52) -> ("Value Expectation"=w48:T2, "Expression"=w32:string, "Expression Check"=w49:T1, "Expectation"=w47:string)
    n192 = Unbundle By Name(w38) -> ("code"=w36:i32)
    n193 = Unbundle By Name(w24) -> ("code"=w37:i32, "source"=w44:string)
    n194 = Not Equal?(x=w36, y=w37) -> (x != y?=w35:bool)
    n195 = call "FTW-ERR-StatusException.vi"("error to check"=w24) -> ("Exception"=w50:T1)
    n196 = Equal?(x=w50, y=w49) -> (x = y?=w45:bool)
    n197 = Equal?(x=w26, y=w48) -> (x = y?=w46:bool)
    n198 = Compound Arithmetic op=AND(w46, w35, w45) -> (w31:bool)
    n199 = Not(x=w31) -> (.not. x?=w30:bool)
    n200 = Bundle("Expression"=w32, "Expression Check"=w49, "Result"=w26, "Expectation"=w47, w31, "source"=w44, "JSON String (UTF-8)"=w22, "Reverse Polish Notation Token Stack"=w25, w42, "Try Paths"=w28) -> (w53:T16)  [unwired: 1 in]
  }
  "Results" <- w10
  "Array" <- w4
  n201 = And Array Elements(Boolean array=w9) -> (logical AND=w8:bool)
  n202 = call "FTW-Regex-Destroy.vi"("Regex"=w11, "error in"=w5) -> ("error out"=w1:errorcluster)  [unwired: 13 in]
  n203 = call "FTW-ERR-Assert-Truthy.vi"("Expected Truthy"=w8, "error in"=w1) -> ("error out"=→"error out":errorcluster)  [unwired: 13 in]
